vi "main.vi"() -> ()   [LabVIEW 2013]
uses:
  states.ctl
  <vilib>/Instr/_visa.llb/VISA Set IO Buffer Mask.ctl
  <resource>/importtools/Common/Event/NISAST Event.lvclass
  <vilib>/Instr/_visa.llb/VISA Configure Serial Port (Instr).vi
panel:
  in  "WaveButt":bool
  in  "机器人编号":enum16{"RoboOne", "RoboTwo"}(ring)
  in  "Run Kinect":bool
  in  "ShowVR":bool
  in  "TCP Port":u16=6001
  out "TCP Error Msg":string
  out "TCP Connection":bool
  out "StopApp":bool
  out "TCP Data":string caption="Data Received from TCP"
  out "TCP Event":bool
  out "StopRobot":bool
  in  "DelayTime":u32=100
  in  "baud rate (9600)":u32=115200 caption="波特率"
  in  "VISA resource name":refnum<visa-resource-name> caption="VISA资源名称"
  out "RoCmdString":string
  in  "StopFour":bool
  in  "ClockWise":bool
  in  "AntiClockWise":bool
  in  "Up":bool
  in  "Down":bool
  in  "StopButton":bool
  in  "States":T1
  # "基于Kinect的机器人控制平台"
  # "COPYRIGHT 2013 Elite Team"
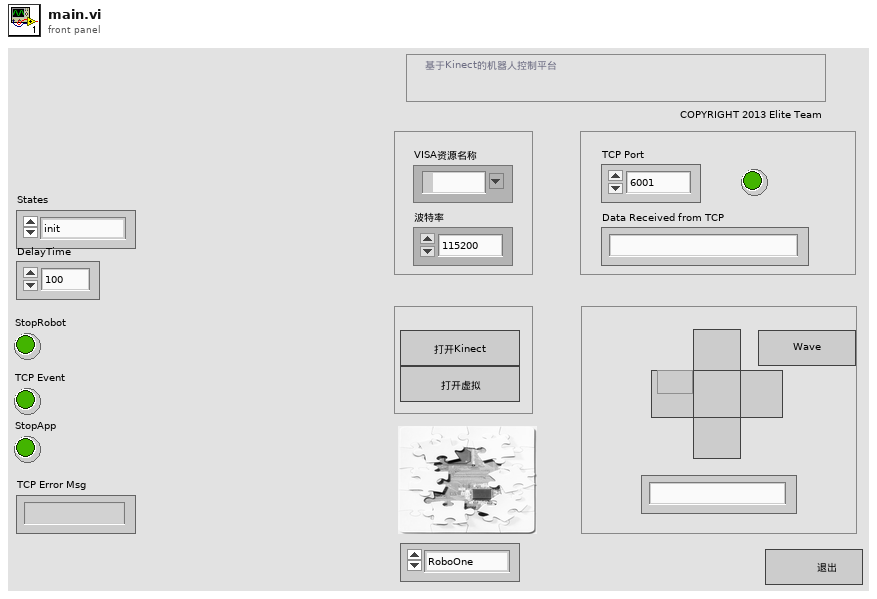
[diagram p1: front panel]
types:
  T1 = typedef "states.ctl" = enum16{"init", "wait", "stop", "ro-up", "ro-down", "ro-clockwise", "ro-anticlockwise", "ro-stopstaut", "ro-wave"}
  T2 = typedef "VISA Set IO Buffer Mask.ctl" = u16
  T3 = enum8{"Enabled", "Disabled", "Disabled and Grayed Out"}
  T4 = enum32{"Invalid", "Standard", "Closed", "Hidden", "Minimized", "Maximized"}
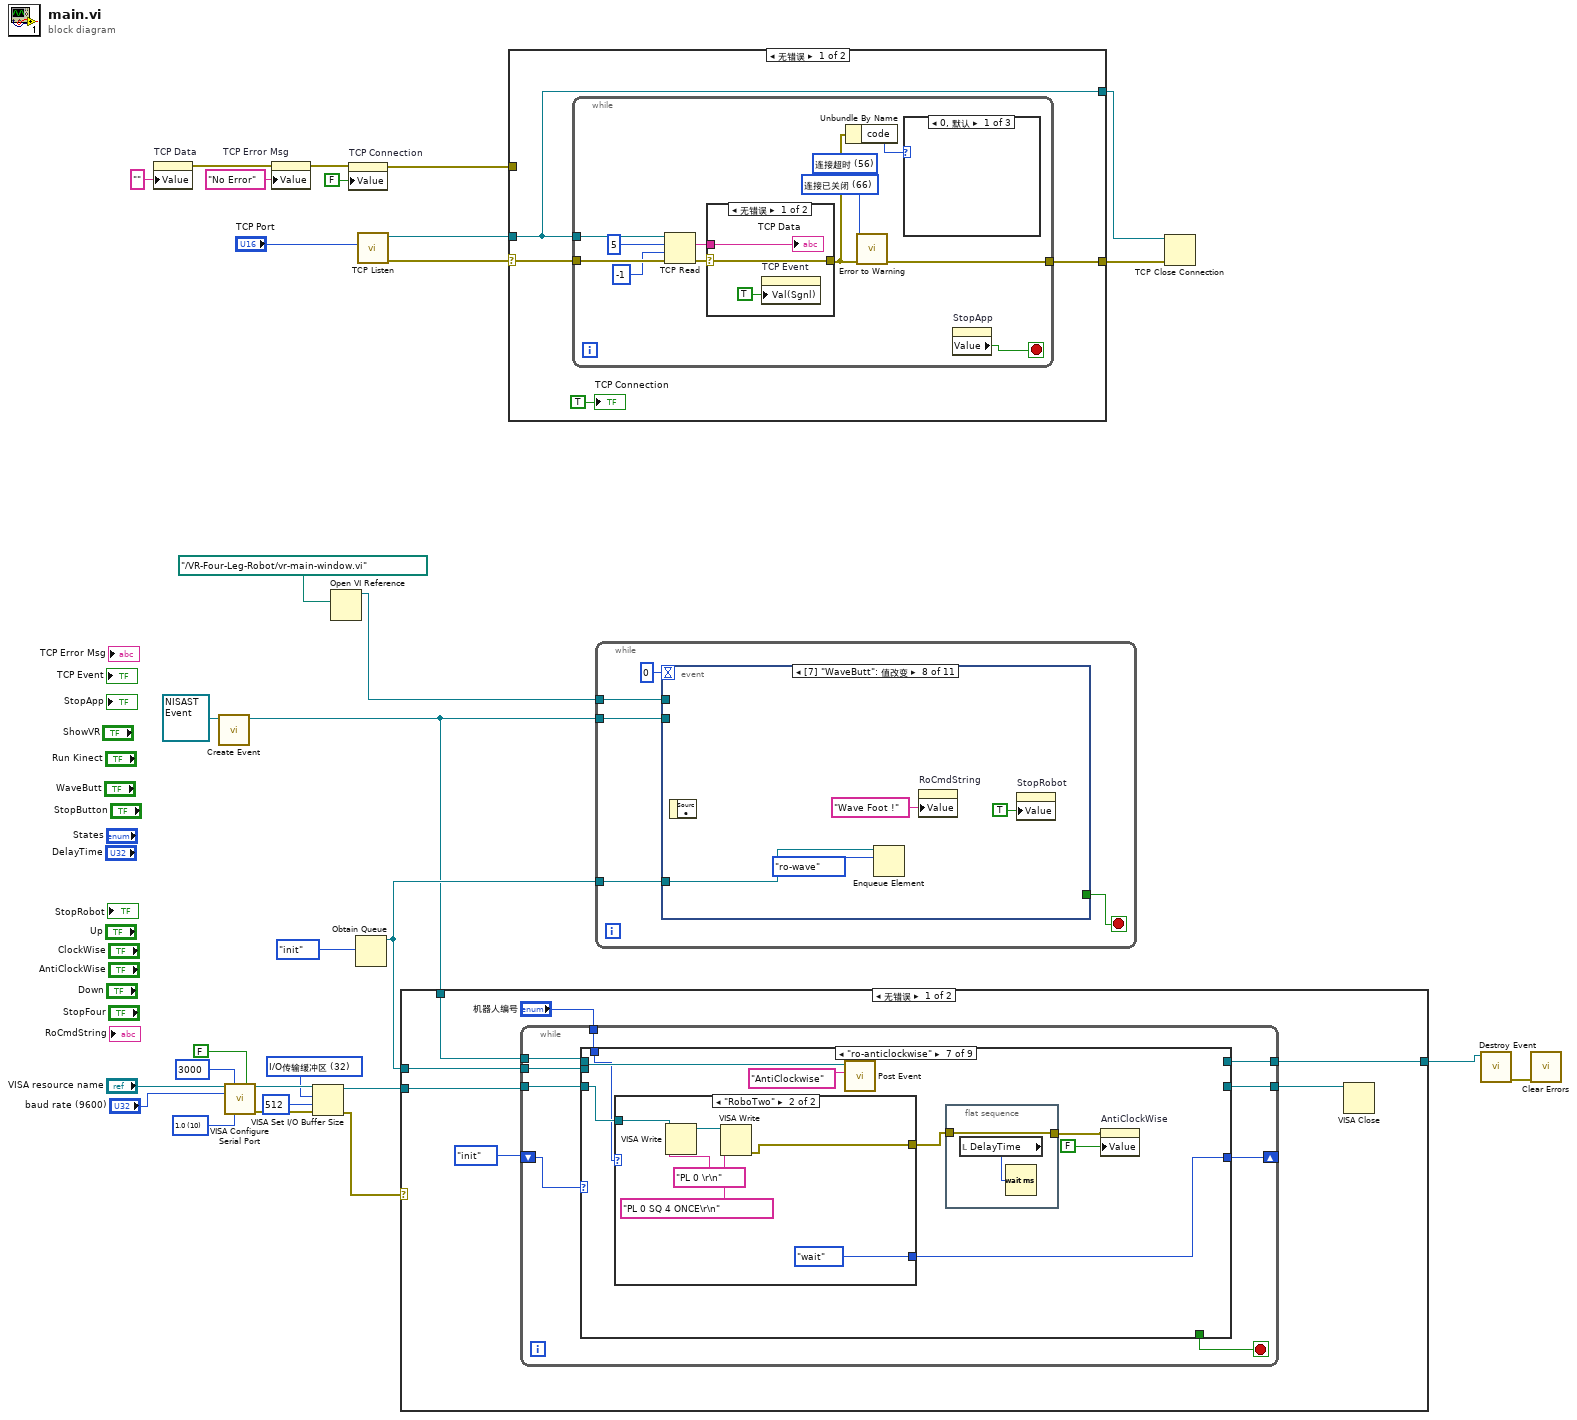
[diagram p0: block diagram]
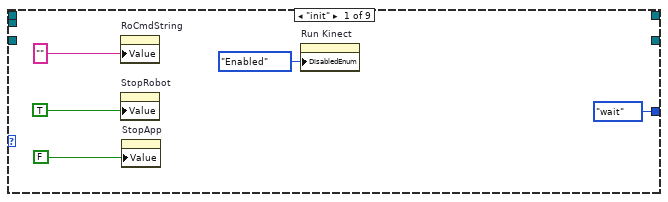
[diagram p2: hidden frame]
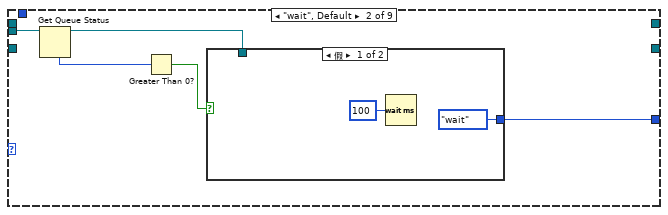
[diagram p3: hidden frame]
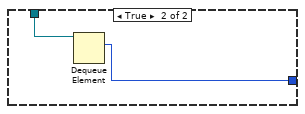
[diagram p4: hidden frame]
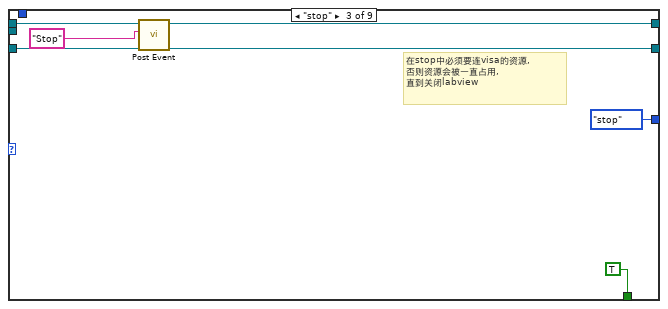
[diagram p5: hidden frame]
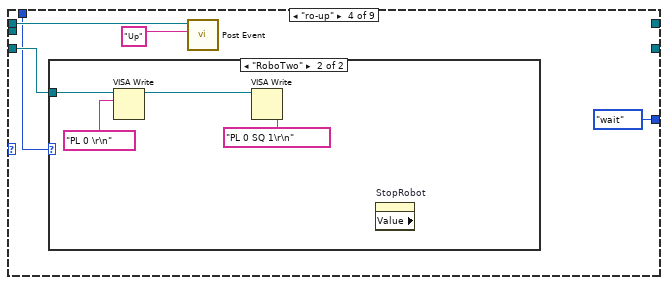
[diagram p6: hidden frame]
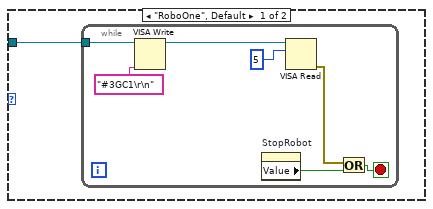
[diagram p7: hidden frame]
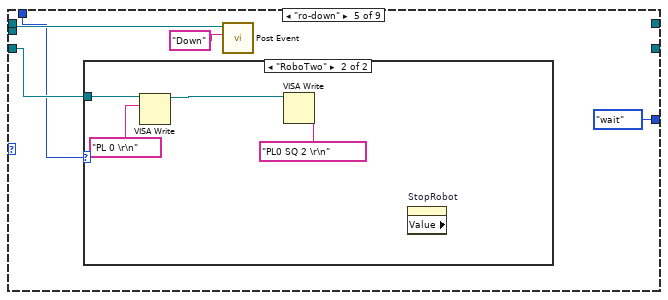
[diagram p8: hidden frame]
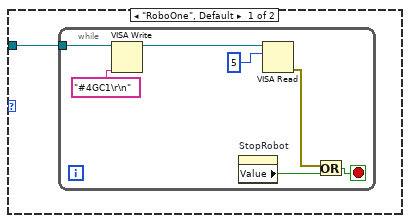
[diagram p9: hidden frame]
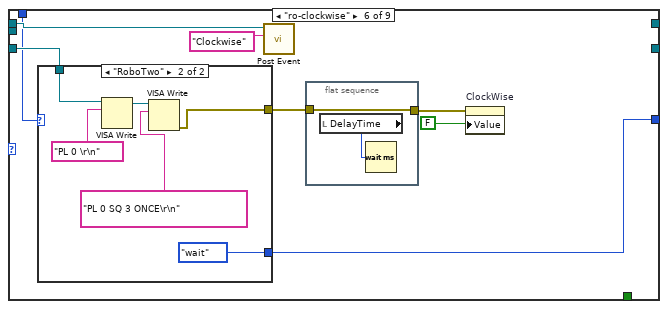
[diagram p10: hidden frame]
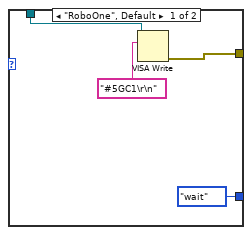
[diagram p11: hidden frame]
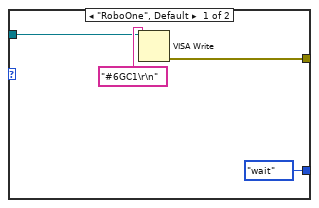
[diagram p12: hidden frame]
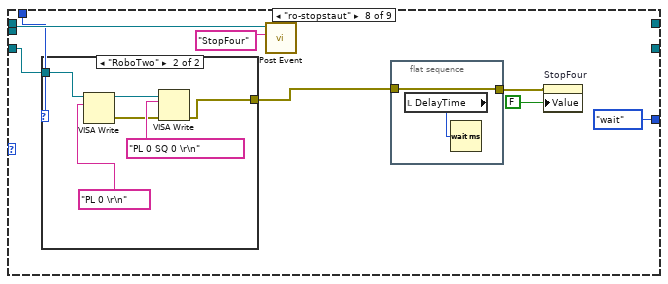
[diagram p13: hidden frame]
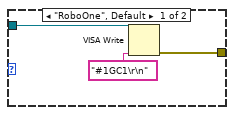
[diagram p14: hidden frame]
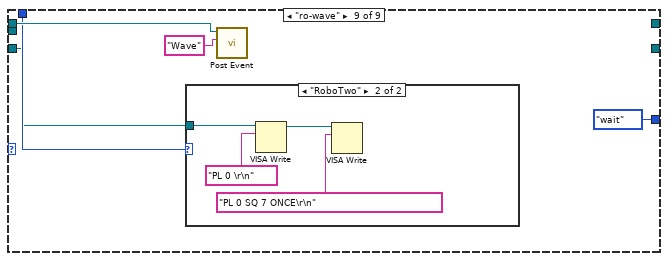
[diagram p15: hidden frame]
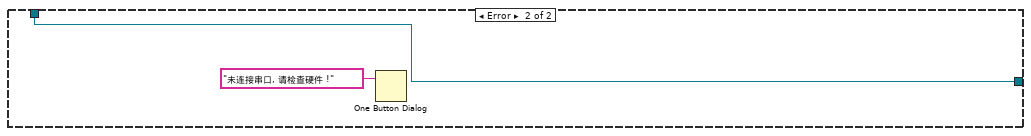
[diagram p17: hidden frame]
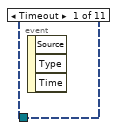
[diagram p18: hidden frame]
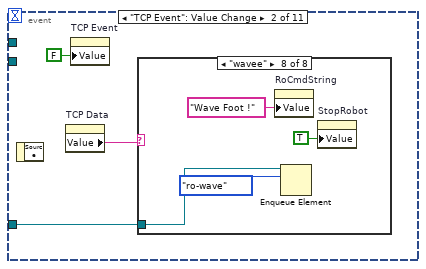
[diagram p19: hidden frame]
diagram:
  w22 = T2 32 items=["I/O接收缓冲区"=16, "I/O传输缓冲区"=32, "I/O接收和传输缓冲区"=48] ("Mask")
  w25 = u16 10 items=["1.0"=10, "1.5"=15, "2.0"=20] ("stop bits (10: 1 bit)")
  n1 = property on="TCP Data" class="Str"("Value"="" ("TCP Data")) -> (error out=w9:errorcluster)  [unwired: 2 in, 1 out]
  n2 = call-dynamic "Create Event.vi"("Event in"=refnum<class "NISAST Event.lvclass"> refnum) -> ("Event out"=w2:refnum<class "NISAST Event.lvclass">)  [unwired: 8 in, 2 out]
  n3 = call-poly "VISA Configure Serial Port"("VISA resource name"="VISA resource name", "timeout (10sec)"=u32 3000, "Enable Termination\nChar (T)"=FALSE ("Enable Termination\nChar (T)"), "baud rate (9600)"="baud rate (9600)", "stop bits (10: 1 bit)"=w25) -> ("VISA resource name out"=w24:refnum<visa-resource-name>, "error out"=w20:errorcluster)  [unwired: 9 in]
  n4 = property on="TCP Error Msg" class="Str"(error in=w9, "Value"="No Error" ("TCP Error Msg")) -> (error out=w10:errorcluster)  [unwired: 1 in, 1 out]
  n5 = VISA Set I/O Buffer Size(VISA resource name=w24, mask (16)=w22, size (4096)=u32 512 ("大小(4096)"), error in (no error)=w20) -> (VISA resource name out=w23:refnum<visa-resource-name>, error out=w5:errorcluster)
  n6 = Open VI Reference(vi path=path "../VR-Four-Leg-Robot/vr-main-window.vi" ("VI路径")) -> (vi reference=w4:refnum<vi>)  [unwired: 5 in, 1 out]
  n7 = property on="TCP Connection" class="Bool (严格)"(error in=w10, "Value"=FALSE ("TCP Connection")) -> (error out=w12:errorcluster)  [unwired: 1 in, 1 out]
  n8 = Obtain Queue(element data type=states."init" ("States")) -> (queue out=w30:refnum<queue>)  [unwired: 4 in, 2 out]
  n9 = call <vilib>:"TCP Listen.vi"("port"="TCP Port") -> ("error out"=w17:errorcluster, "connection ID"=w16:refnum<k5>)  [unwired: 6 in, 3 out]
  n10 = case shown="无错误" w5 {
    tunnel: w30 -> [w37 _]
    tunnel: w23 -> [w34 _]
    tunnel: w2 -> [w33 w169]
    tunnel: [w32 w169] -> w1
    frame No Error {
      n11 = while {
        tunnel: w37 -> [w44]
        shift-right: [w43] -> _
        shift-left: states."init" ("States") -> [w46]
        tunnel: w34 -> [w42]
        tunnel: [w41] -> w35
        tunnel: w33 -> [w40]
        tunnel: [w39] -> w32
        tunnel: "机器人编号" -> [w38]
        stop <- w45 stop-if-true
        n12 = case shown="\"ro-anticlockwise\"" w46 {
          tunnel: [_ _ TRUE _ _ _ _ _ _] -> w45
          tunnel: w44 -> [_ w56 _ _ _ _ _ _ _]
          tunnel: [states."wait" ("States") w52 states."stop" ("States") states."wait" ("States") states."wait" ("States") w101 w121 states."wait" ("States") states."wait" ("States")] -> w43
          tunnel: w42 -> [_ _ w64 w70 w87 w108 w128 w148 w160]
          tunnel: [_ _ w64 _ _ _ _ _ _] -> w41
          tunnel: w40 -> [_ _ w62 w68 w85 w103 w123 w142 w164]
          tunnel: [_ _ w61 _ _ _ _ _ _] -> w39
          tunnel: w38 -> [_ _ _ w67 w84 w102 w122 w141 w161]
          frame "init" {
            n13 = property on="RoCmdString" class="Str"("Value"="" ("RoCmdString")) -> ()  [unwired: 2 in, 2 out]
            n14 = property on="StopRobot" class="Bool (严格)"("Value"=TRUE ("StopRobot")) -> ()  [unwired: 2 in, 2 out]
            n15 = property on="StopApp" class="Bool (严格)"("Value"=FALSE ("StopApp")) -> ()  [unwired: 2 in, 2 out]
            n16 = property on="Run Kinect" class="Bool"("DisabledEnum"=T3."Enabled" ("禁用")) -> ()  [unwired: 2 in, 2 out]
          }
          frame "wait", Default {
            n17 = Get Queue Status(queue=w56) -> (queue out=w53:refnum<queue>, # elements in queue=w55:i32)  [unwired: 2 in, 6 out]
            n18 = Greater Than 0?(x=w55) -> (x > 0?=w54:bool)
            n19 = case shown="假" w54 {
              tunnel: w53 -> [_ w60]
              tunnel: [states."wait" ("States") w59] -> w52
              frame False {
                n20 = Wait (ms)(milliseconds to wait=u32 100 ("等待时间（毫秒）")) -> ()  [unwired: 1 out]
              }
              frame True {
                n21 = Dequeue Element(queue=w60) -> (element=w59:T1)  [unwired: 2 in, 3 out]
              }
            }
          }
          frame "stop" {
            # "在stop中必须要连visa的资源,\n否则资源会被一直占用,\n直到关闭labview"
            n22 = call-dynamic "Post Event.vi"("Event Name"="Stop", "Event in"=w62) -> ("Event out"=w61:refnum<class "NISAST Event.lvclass">)  [unwired: 8 in, 1 out]
          }
          frame "ro-up" {
            n23 = case shown="\"RoboTwo\"" w67 {
              tunnel: w70 -> [w72 w82]
              frame "RoboOne", Default {
                n24 = while {
                  tunnel: w72 -> [w78]
                  stop <- w73 stop-if-true
                  n25 = VISA Write(VISA resource name=w78, write buffer="#3GC1\r\n" ("写入缓冲区")) -> (VISA resource name out=w76:refnum<visa-resource-name>)  [unwired: 1 in, 2 out]
                  n26 = property on="StopRobot" class="Bool (严格)"() -> ("Value"=w74:bool)  [unwired: 2 in, 2 out]
                  n27 = VISA Read(VISA resource name=w76, byte count=u32 5 ("字节总数")) -> (error out=w75:errorcluster)  [unwired: 1 in, 3 out]
                  n28 = Or(x=w75, y=w74) -> (x .or. y?=w73:bool)
                }
              }
              frame "RoboTwo" {
                n29 = VISA Write(VISA resource name=w82, write buffer="PL 0 \r\n" ("写入缓冲区")) -> (VISA resource name out=w81:refnum<visa-resource-name>)  [unwired: 1 in, 2 out]
                n30 = VISA Write(VISA resource name=w81, write buffer="PL 0 SQ 1\r\n" ("写入缓冲区")) -> ()  [unwired: 1 in, 3 out]
                n31 = property on="StopRobot" class="Bool (严格)" props=["Value"]() -> ()  [unwired: 2 in, 3 out]
              }
            }
            n32 = call-dynamic "Post Event.vi"("Event Name"="Up", "Event in"=w68) -> ()  [unwired: 8 in, 2 out]
          }
          frame "ro-down" {
            n33 = case shown="\"RoboTwo\"" w84 {
              tunnel: w87 -> [w89 w99]
              frame "RoboOne", Default {
                n34 = while {
                  tunnel: w89 -> [w95]
                  stop <- w90 stop-if-true
                  n35 = VISA Write(VISA resource name=w95, write buffer="#4GC1\r\n" ("写入缓冲区")) -> (VISA resource name out=w93:refnum<visa-resource-name>)  [unwired: 1 in, 2 out]
                  n36 = property on="StopRobot" class="Bool (严格)"() -> ("Value"=w91:bool)  [unwired: 2 in, 2 out]
                  n37 = VISA Read(VISA resource name=w93, byte count=u32 5 ("字节总数")) -> (error out=w92:errorcluster)  [unwired: 1 in, 3 out]
                  n38 = Or(x=w92, y=w91) -> (x .or. y?=w90:bool)
                }
              }
              frame "RoboTwo" {
                n39 = VISA Write(VISA resource name=w99, write buffer="PL 0 \r\n" ("写入缓冲区")) -> (VISA resource name out=w98:refnum<visa-resource-name>)  [unwired: 1 in, 2 out]
                n40 = VISA Write(VISA resource name=w98, write buffer="PL0 SQ 2 \r\n" ("写入缓冲区")) -> ()  [unwired: 1 in, 3 out]
                n41 = property on="StopRobot" class="Bool (严格)" props=["Value"]() -> ()  [unwired: 2 in, 3 out]
              }
            }
            n42 = call-dynamic "Post Event.vi"("Event Name"="Down", "Event in"=w85) -> ()  [unwired: 8 in, 2 out]
          }
          frame "ro-clockwise" {
            n43 = case shown="\"RoboTwo\"" w102 {
              tunnel: w108 -> [w111 w118]
              tunnel: [w110 w113] -> w106
              tunnel: [states."wait" ("States") states."wait" ("States")] -> w101
              frame "RoboOne", Default {
                n44 = VISA Write(VISA resource name=w111, write buffer="#5GC1\r\n" ("写入缓冲区")) -> (error out=w110:errorcluster)  [unwired: 1 in, 2 out]
              }
              frame "RoboTwo" {
                n45 = VISA Write(VISA resource name=w118, write buffer="PL 0 \r\n" ("写入缓冲区")) -> (VISA resource name out=w117:refnum<visa-resource-name>)  [unwired: 1 in, 2 out]
                n46 = VISA Write(VISA resource name=w117, write buffer="PL 0 SQ 3 ONCE\r\n" ("写入缓冲区")) -> (error out=w113:errorcluster)  [unwired: 1 in, 2 out]
              }
            }
            n47 = call-dynamic "Post Event.vi"("Event Name"="Clockwise", "Event in"=w103) -> ()  [unwired: 8 in, 2 out]
            n48 = flat-sequence {
              tunnel: [w120] -> w107
              tunnel: w106 -> [w120]
              frame #0 {
                n49 = local read "DelayTime"() -> (w119:u32)
                n50 = Wait (ms)(milliseconds to wait=w119) -> ()  [unwired: 1 out]
              }
            }
            n51 = property on="ClockWise" class="Bool (严格)"(error in=w107, "Value"=FALSE ("Up")) -> ()  [unwired: 1 in, 2 out]
          }
          frame "ro-anticlockwise" {
            n52 = case shown="\"RoboTwo\"" w122 {
              tunnel: w128 -> [w131 w138]
              tunnel: [w130 w133] -> w125
              tunnel: [states."wait" ("States") states."wait" ("States")] -> w121
              frame "RoboOne", Default {
                n53 = VISA Write(VISA resource name=w131, write buffer="#6GC1\r\n" ("写入缓冲区")) -> (error out=w130:errorcluster)  [unwired: 1 in, 2 out]
              }
              frame "RoboTwo" {
                n54 = VISA Write(VISA resource name=w138, write buffer="PL 0 \r\n" ("写入缓冲区")) -> (VISA resource name out=w137:refnum<visa-resource-name>)  [unwired: 1 in, 2 out]
                n55 = VISA Write(VISA resource name=w137, write buffer="PL 0 SQ 4 ONCE\r\n" ("写入缓冲区")) -> (error out=w133:errorcluster)  [unwired: 1 in, 2 out]
              }
            }
            n56 = call-dynamic "Post Event.vi"("Event Name"="AntiClockwise", "Event in"=w123) -> ()  [unwired: 8 in, 2 out]
            n57 = flat-sequence {
              tunnel: [w140] -> w126
              tunnel: w125 -> [w140]
              frame #0 {
                n58 = local read "DelayTime"() -> (w139:u32)
                n59 = Wait (ms)(milliseconds to wait=w139) -> ()  [unwired: 1 out]
              }
            }
            n60 = property on="AntiClockWise" class="Bool (严格)"(error in=w126, "Value"=FALSE ("Up")) -> ()  [unwired: 1 in, 2 out]
          }
          frame "ro-stopstaut" {
            n61 = case shown="\"RoboTwo\"" w141 {
              tunnel: w148 -> [w150 w155]
              tunnel: [w149 w157] -> w144
              frame "RoboOne", Default {
                n62 = VISA Write(VISA resource name=w150, write buffer="#1GC1\r\n" ("写入缓冲区")) -> (error out=w149:errorcluster)  [unwired: 1 in, 2 out]
              }
              frame "RoboTwo" {
                n63 = VISA Write(VISA resource name=w155, write buffer="PL 0 \r\n" ("写入缓冲区")) -> (VISA resource name out=w154:refnum<visa-resource-name>, error out=w153:errorcluster)  [unwired: 1 in, 1 out]
                n64 = VISA Write(VISA resource name=w154, write buffer="PL 0 SQ 0 \r\n" ("写入缓冲区"), error in (no error)=w153) -> (error out=w157:errorcluster)  [unwired: 2 out]
              }
            }
            n65 = call-dynamic "Post Event.vi"("Event Name"="StopFour", "Event in"=w142) -> ()  [unwired: 8 in, 2 out]
            n66 = flat-sequence {
              tunnel: [w159] -> w146
              tunnel: w144 -> [w159]
              frame #0 {
                n67 = local read "DelayTime"() -> (w158:u32)
                n68 = Wait (ms)(milliseconds to wait=w158) -> ()  [unwired: 1 out]
              }
            }
            n69 = property on="StopFour" class="Bool (严格)"(error in=w146, "Value"=FALSE ("Up")) -> ()  [unwired: 1 in, 2 out]
          }
          frame "ro-wave" {
            n70 = case shown="\"RoboTwo\"" w161 {
              tunnel: w160 -> [_ w168]
              frame "RoboOne", Default {
              }
              frame "RoboTwo" {
                n71 = VISA Write(VISA resource name=w168, write buffer="PL 0 \r\n" ("写入缓冲区")) -> (VISA resource name out=w167:refnum<visa-resource-name>)  [unwired: 1 in, 2 out]
                n72 = VISA Write(VISA resource name=w167, write buffer="PL 0 SQ 7 ONCE\r\n" ("写入缓冲区")) -> ()  [unwired: 1 in, 3 out]
              }
            }
            n73 = call-dynamic "Post Event.vi"("Event Name"="Wave", "Event in"=w164) -> ()  [unwired: 8 in, 2 out]
          }
        }
      }
      n74 = VISA Close(VISA resource name=w35) -> ()  [unwired: 1 in, 1 out]
    }
    frame Error {
      n75 = One Button Dialog(message="未连接串口, 请检查硬件 !" ("消息")) -> ()  [unwired: 1 in, 1 out]
    }
  }
  n76 = case shown="无错误" w17 {
    selector: w17 -> [w174 w193]
    tunnel: w16 -> [w172 w194]
    tunnel: [w173 w193] -> w15
    tunnel: [w172 w194] -> w14
    tunnel: w12 -> [_ _]
    frame No Error {
      n77 = while {
        tunnel: w172 -> [w186]
        tunnel: w174 -> [w185]
        tunnel: [w177] -> w173
        stop <- w178 stop-if-true
        w182 = 66 items=["无错误", "参数错误", "内存已满", "超出区域", "文件结束", "文件已打开", "一般文件IO错误", "未找到文件", "文件权限错误", "磁盘已满", "路径副本", "打开过多文件", "未启用", "未找到资源文件", "无法添加资源", "未找到资源", "未找到图像", "图像内存错误", "画笔不存在", "配置错误类型", "配置未找到解析段", "配置解析错误", "配置内存错误", "错误外部代码格式", "错误外部代码偏移量", "外部代码不存在", "空窗口", "销毁窗口错误", "空菜单", "打印已中止", "错误打印记录", "打印驱动程序错误", "打印时窗口错误", "打印时内存错误", "打印对话框错误", "一般打印错误", "无效设备引用句柄", "设备未找到", "设备参数错误", "设备单位错误", "无法打开设备", "设备调用已中止", "一般错误", "用户已取消", "对象ID过低", "对象ID过高", "对象不在堆中", "未知的堆", "错误DefProc ID", "DefProc不在表格中", "范围外信息", "空方法", "未知信息", "不支持管理器调用", "错误地址", "连接过程中", "连接超时", "连接过程中", "不支持网络属性", "网络错误", "正在使用的地址", "系统缺少内存", "连接已中止", "连接已拒绝", "连接未建立", "连接已建立", "连接已关闭", "初始化错误（交互应用程序管理器）", "错误事件发生", "等待无约束事件发生处理程序", "事件发生队列溢出", "错误路径", "未发出信号量", "未识别类型（交互应用程序管理器）"] ("2nd Error to Convert")
        w181 = 56 items=["无错误", "参数错误", "内存已满", "超出区域", "文件结束", "文件已打开", "一般文件IO错误", "未找到文件", "文件权限错误", "磁盘已满", "路径副本", "打开过多文件", "未启用", "未找到资源文件", "无法添加资源", "未找到资源", "未找到图像", "图像内存错误", "画笔不存在", "配置错误类型", "配置未找到解析段", "配置解析错误", "配置内存错误", "错误外部代码格式", "错误外部代码偏移量", "外部代码不存在", "空窗口", "销毁窗口错误", "空菜单", "打印已中止", "错误打印记录", "打印驱动程序错误", "打印时窗口错误", "打印时内存错误", "打印对话框错误", "一般打印错误", "无效设备引用句柄", "设备未找到", "设备参数错误", "设备单位错误", "无法打开设备", "设备调用已中止", "一般错误", "用户已取消", "对象ID过低", "对象ID过高", "对象不在堆中", "未知的堆", "错误DefProc ID", "DefProc不在表格中", "范围外信息", "空方法", "未知信息", "不支持管理器调用", "错误地址", "连接过程中", "连接超时", "连接过程中", "不支持网络属性", "网络错误", "正在使用的地址", "系统缺少内存", "连接已中止", "连接已拒绝", "连接未建立", "连接已建立", "连接已关闭", "初始化错误（交互应用程序管理器）", "错误事件发生", "等待无约束事件发生处理程序", "事件发生队列溢出", "错误路径", "未发出信号量", "未识别类型（交互应用程序管理器）"] ("1st Error to Convert")
        n78 = TCP Read(connection ID=w186, bytes to read=5 ("读取的字节"), error in (no error)=w185, 9:-1 ("超时毫秒(25000)")) -> (data out=w179:string, error out=w180:errorcluster)  [unwired: 2 out]
        n79 = case shown="无错误" w180 {
          selector: w180 -> [w190 w192]
          tunnel: w179 -> [w191 _]
          tunnel: [w190 w192] -> w175
          frame No Error {
            n80 = property on="TCP Event" class="Bool (严格)"("Val(Sgnl)"=TRUE ("值(信号)")) -> ()  [unwired: 2 in, 2 out]
            "TCP Data" <- w191
          }
          frame Error {
          }
        }
        n81 = Unbundle By Name(w175) -> ("code"=w176:i32)
        n82 = call <vilib>:"Error to Warning.vi"("1st Error to Convert"=w181, "2nd Error to Convert"=w182, "error in"=w175) -> ("warning out"=w177:errorcluster)  [unwired: 12 in]
        n83 = case shown="0, 默认" w176 {
          frame 0, Default {
          }
          frame 66 {
            n84 = property on="TCP Error Msg" class="Str"("Value"="连接已关闭" ("TCP Error Msg")) -> ()  [unwired: 2 in, 2 out]
          }
          frame 56 {
            n85 = property on="TCP Error Msg" class="Str"("Value"="连接超时" ("TCP Error Msg")) -> ()  [unwired: 2 in, 2 out]
          }
        }
        n86 = property on="StopApp" class="Bool (严格)"() -> ("Value"=w178:bool)  [unwired: 2 in, 2 out]
      }
      "TCP Connection" <- TRUE ("TCP Connection")
    }
    frame Error {
    }
  }
  n87 = while {
    tunnel: w30 -> [w199]
    tunnel: w2 -> [w195]
    tunnel: w4 -> [w196]
    stop <- w198 stop-if-true
    n88 = event shown="[7] \"WaveButt\": 值改变" {
      selector: _ -> [_ _ _ _ _ _ _ _ _ _ _]
      dyn-events: _ -> [_ _ _ _ _ _ _ _ _ _ _]
      timeout: 0 -> [_ _ _ _ _ _ _ _ _ _ _]
      tunnel: w199 -> [_ w201 w229 w236 w240 w244 w248 w250 w255 _ _]
      tunnel: [_ _ TRUE _ _ _ _ _ _ _ _] -> w198
      tunnel: w196 -> [_ _ _ _ _ _ _ _ _ w260 _]
      tunnel: w195 -> [_ _ _ _ _ _ _ _ _ w258 _]
      event Timeout {
        n89 = event-data() -> ()  [unwired: 1 in, 3 out]
      }
      event "TCP Event": Value Change {
        n90 = event-data() -> ()  [unwired: 1 in, 1 out]
        n91 = property on="TCP Data" class="Str"() -> ("Value"=w200:string)  [unwired: 2 in, 2 out]
        n92 = property on="TCP Event" class="Bool (严格)"("Value"=FALSE ("TCP Event")) -> ()  [unwired: 2 in, 2 out]
        n93 = case shown="\"wavee\"" w200 {
          tunnel: w201 -> [_ w203 w207 w211 w215 w219 _ w223]
          frame "testt", Default {
          }
          frame "gogog" {
            # "up"
            n94 = property on="StopRobot" class="Bool (严格)"("Value"=FALSE ("StopRobot")) -> ()  [unwired: 2 in, 2 out]
            n95 = property on="RoCmdString" class="Str"("Value"="Go Up !" ("RoCmdString")) -> ()  [unwired: 2 in, 2 out]
            n96 = Enqueue Element(queue=w203, element=states."ro-up" ("States")) -> ()  [unwired: 2 in, 3 out]
          }
          frame "backk" {
            n97 = property on="RoCmdString" class="Str"("Value"="Go Down !" ("RoCmdString")) -> ()  [unwired: 2 in, 2 out]
            n98 = Enqueue Element(queue=w207, element=states."ro-down" ("States")) -> ()  [unwired: 2 in, 3 out]
            n99 = property on="StopRobot" class="Bool (严格)"("Value"=FALSE ("StopRobot")) -> ()  [unwired: 2 in, 2 out]
          }
          frame "stopp" {
            n100 = property on="RoCmdString" class="Str"("Value"="Stop Staut !" ("RoCmdString")) -> ()  [unwired: 2 in, 2 out]
            n101 = Enqueue Element(queue=w211, element=states."ro-stopstaut" ("States")) -> ()  [unwired: 2 in, 3 out]
            n102 = property on="StopRobot" class="Bool (严格)"("Value"=TRUE ("StopRobot")) -> ()  [unwired: 2 in, 2 out]
          }
          frame "leftt" {
            n103 = property on="RoCmdString" class="Str"("Value"="Turn Anticlockwise !" ("RoCmdString")) -> ()  [unwired: 2 in, 2 out]
            n104 = property on="StopRobot" class="Bool (严格)"("Value"=TRUE ("StopRobot")) -> ()  [unwired: 2 in, 2 out]
            n105 = Enqueue Element(queue=w215, element=states."ro-anticlockwise" ("States")) -> ()  [unwired: 2 in, 3 out]
          }
          frame "right" {
            n106 = property on="RoCmdString" class="Str"("Value"="Turn Clockwise !" ("RoCmdString")) -> ()  [unwired: 2 in, 2 out]
            n107 = Enqueue Element(queue=w219, element=states."ro-clockwise" ("States")) -> ()  [unwired: 2 in, 3 out]
            n108 = property on="StopRobot" class="Bool (严格)"("Value"=TRUE ("StopRobot")) -> ()  [unwired: 2 in, 2 out]
          }
          frame "nonee" {
          }
          frame "wavee" {
            n109 = property on="RoCmdString" class="Str"("Value"="Wave Foot !" ("RoCmdString")) -> ()  [unwired: 2 in, 2 out]
            n110 = Enqueue Element(queue=w223, element=states."ro-wave" ("States")) -> ()  [unwired: 2 in, 3 out]
            n111 = property on="StopRobot" class="Bool (严格)"("Value"=TRUE ("StopRobot")) -> ()  [unwired: 2 in, 2 out]
          }
        }
      }
      event "StopButton": Value Change {
        n112 = event-data() -> ()  [unwired: 1 in, 1 out]
        n113 = Enqueue Element(queue=w229, element=states."ro-stopstaut" ("States")) -> (queue out=w228:refnum<queue>)  [unwired: 2 in, 2 out]
        n114 = Enqueue Element(queue=w228, element=states."stop" ("States")) -> ()  [unwired: 2 in, 3 out]
        n115 = property on="StopApp" class="Bool (严格)"("Value"=TRUE ("StopApp")) -> ()  [unwired: 2 in, 2 out]
        n116 = property on="StopRobot" class="Bool (严格)"("Value"=TRUE ("StopRobot")) -> ()  [unwired: 2 in, 2 out]
      }
      event "Up": Value Change {
        n117 = event-data() -> ()  [unwired: 1 in, 2 out]
        n118 = property on="RoCmdString" class="Str"("Value"="Go Up !" ("RoCmdString")) -> ()  [unwired: 2 in, 2 out]
        n119 = Enqueue Element(queue=w236, element=states."ro-up" ("States")) -> ()  [unwired: 2 in, 3 out]
        n120 = property on="StopRobot" class="Bool (严格)"("Value"=FALSE ("StopRobot")) -> ()  [unwired: 2 in, 2 out]
      }
      event "Down": Value Change {
        n121 = event-data() -> ()  [unwired: 1 in, 5 out]
        n122 = Enqueue Element(queue=w240, element=states."ro-down" ("States")) -> ()  [unwired: 2 in, 3 out]
        n123 = property on="RoCmdString" class="Str"("Value"="Go Down !" ("RoCmdString")) -> ()  [unwired: 2 in, 2 out]
        n124 = property on="StopRobot" class="Bool (严格)"("Value"=FALSE ("StopRobot")) -> ()  [unwired: 2 in, 2 out]
      }
      event "ClockWise": Value Change {
        n125 = event-data() -> ()  [unwired: 1 in, 5 out]
        n126 = Enqueue Element(queue=w244, element=states."ro-clockwise" ("States")) -> ()  [unwired: 2 in, 3 out]
        n127 = property on="RoCmdString" class="Str"("Value"="Turn Clockwise !" ("RoCmdString")) -> ()  [unwired: 2 in, 2 out]
        n128 = property on="StopRobot" class="Bool (严格)"("Value"=TRUE ("StopRobot")) -> ()  [unwired: 2 in, 2 out]
      }
      event "AntiClockWise": Value Change {
        n129 = event-data() -> ()  [unwired: 1 in, 1 out]
        n130 = Enqueue Element(queue=w248, element=states."ro-anticlockwise" ("States")) -> ()  [unwired: 2 in, 3 out]
        n131 = property on="RoCmdString" class="Str"("Value"="Turn Anticlockwise !" ("RoCmdString")) -> ()  [unwired: 2 in, 2 out]
        n132 = property on="StopRobot" class="Bool (严格)"("Value"=TRUE ("StopRobot")) -> ()  [unwired: 2 in, 2 out]
      }
      event "WaveButt": Value Change {
        n133 = event-data() -> ()  [unwired: 1 in, 1 out]
        n134 = Enqueue Element(queue=w250, element=states."ro-wave" ("States")) -> ()  [unwired: 2 in, 3 out]
        n135 = property on="RoCmdString" class="Str"("Value"="Wave Foot !" ("RoCmdString")) -> ()  [unwired: 2 in, 2 out]
        n136 = property on="StopRobot" class="Bool (严格)"("Value"=TRUE ("StopRobot")) -> ()  [unwired: 2 in, 2 out]
      }
      event "StopFour": Value Change {
        n137 = event-data() -> ()  [unwired: 1 in, 5 out]
        n138 = Enqueue Element(queue=w255, element=states."ro-stopstaut" ("States")) -> ()  [unwired: 2 in, 3 out]
        n139 = property on="RoCmdString" class="Str"("Value"="Stop Staut !" ("RoCmdString")) -> ()  [unwired: 2 in, 2 out]
        n140 = property on="StopRobot" class="Bool (严格)"("Value"=TRUE ("StopRobot")) -> ()  [unwired: 2 in, 2 out]
      }
      event "ShowVR": Value Change {
        n141 = event-data() -> ("NewVal"=w259:bool)  [unwired: 1 in]
        n142 = case shown="真" w259 {
          tunnel: w260 -> [_ w264]
          tunnel: w258 -> [w261 w263]
          frame False {
            n143 = call-dynamic "Post Event.vi"("Event Name"="Stop", "Event in"=w261) -> ()  [unwired: 8 in, 2 out]
          }
          frame True {
            n144 = invoke class="VI" method="Ctrl Val.Set"(reference=w264, "Control Name"="EventIn" ("控件名"), "Value"=w263) -> (reference out=w266:refnum<vi>, error out=w267:errorcluster)  [unwired: 2 in, 3 out]
            n145 = invoke class="VI" method="FP.Open"(reference=w266, error in=w267, "State"=T4."Hidden" ("状态")) -> (reference out=w268:refnum<vi>, error out=w269:errorcluster)  [unwired: 2 in, 3 out]
            n146 = invoke class="VI" method="Run VI"(reference=w268, error in=w269, "Wait until done"=FALSE ("结束前等待")) -> ()  [unwired: 2 in, 5 out]
          }
        }
      }
      event "Run Kinect": Value Change {
        n147 = event-data() -> ()  [unwired: 1 in, 1 out]
        n148 = call "execute-exe.vi"() -> ()  [unwired: 10 in, 2 out]
        n149 = property on="Run Kinect" class="Bool"("DisabledEnum"=T3."Disabled and Grayed Out" ("禁用")) -> ()  [unwired: 2 in, 2 out]
      }
    }
  }
  n150 = TCP Close Connection(connection ID=w14, error in (no error)=w15) -> ()  [unwired: 1 in, 2 out]
  n151 = call-dynamic "Destroy Event.vi"("Event in"=w1) -> ("error out"=w3:errorcluster)  [unwired: 9 in, 1 out]
  n152 = call <vilib>:"Clear Errors.vi"("error in (no error)"=w3) -> ()  [unwired: 6 in, 1 out]
